vi "Write DeviceDataModel[].vi"(8 "error in (no error)":errorcluster caption="错误输入（无错误）", 10 "DeviceDataModel[]":refnum<data-value>, 11 "Super Data Model输入":refnum<class "Super Data Model.lvclass">) -> (0 "error out":errorcluster caption="错误输出", 3 "Super Data Model输出":refnum<class "Super Data Model.lvclass">)   [LabVIEW 2013, in "Modbus Library - Advance.lvlib" / "Super Data Model.lvclass"]
uses:
  Super Data Model.lvclass
  Standard Data Model/Standard Data Model.lvclass
  Super Data Model.lvclass/Super Data Model.ctl
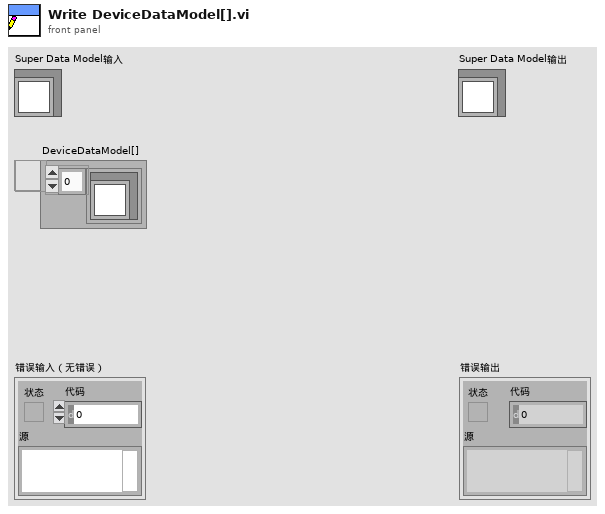
[diagram p1: front panel]
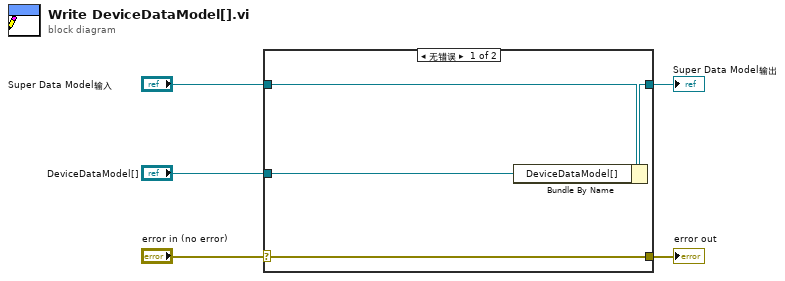
[diagram p0: block diagram]
diagram:
  n1 = case shown="无错误" "error in (no error)" {
    selector: "error in (no error)" -> [w9 w10]
    tunnel: [w9 w10] -> w4
    tunnel: [w7 w11] -> w2
    tunnel: "Super Data Model输入" -> [w8 w11]
    tunnel: "DeviceDataModel[]" -> [w6 _]
    frame No Error {
      n2 = Bundle By Name(cluster=w8, "DeviceDataModel[]"=w6) -> (w7:refnum<class "Super Data Model.lvclass">)
    }
    frame Error {
    }
  }
  "error out" <- w4
  "Super Data Model输出" <- w2
